vi "set_S12CON.vi"(8 "error in (no error)":errorcluster caption="错误输入（无错误）", 9 "S12CON寄存器设置":T1={"S2传感器上升沿绑定动作"=0, "S2传感器下降沿绑定动作"=1, "S1传感器上升沿绑定动作"=2, "S1传感器下降沿绑定动作"=3} {"S1传感器下降沿绑定动作" items=["无动作，无状态通知"=0, "无动作，有通知"=1, "负向连续运行"=2, "减速直到停止"=3, "紧急停止"=4, "负向相对位移控制"=5, "绝对位置清零"=6, "绝对位置清零+相对位移控制"=7, "换向相对位移控制"=9, "正向连续运行"=10, "绝对位置清零+减速直到停止"=11, "绝对位置清零+紧急停止"=12, "正向相对位移控制"=13, "换向连续运行"=14, "脱机"=15]; "S1传感器上升沿绑定动作" items=["无动作，无状态通知"=0, "无动作，有通知"=1, "负向连续运行"=2, "减速直到停止"=3, "紧急停止"=4, "负向相对位移控制"=5, "绝对位置清零"=6, "绝对位置清零+相对位移控制"=7, "换向相对位移控制"=9, "正向连续运行"=10, "绝对位置清零+减速直到停止"=11, "绝对位置清零+紧急停止"=12, "正向相对位移控制"=13, "换向连续运行"=14, "脱机"=15]; "S2传感器下降沿绑定动作" items=["无动作，无状态通知"=0, "无动作，有通知"=1, "负向连续运行"=2, "减速直到停止"=3, "紧急停止"=4, "负向相对位移控制"=5, "绝对位置清零"=6, "绝对位置清零+相对位移控制"=7, "换向相对位移控制"=9, "正向连续运行"=10, "绝对位置清零+减速直到停止"=11, "绝对位置清零+紧急停止"=12, "正向相对位移控制"=13, "换向连续运行"=14, "脱机"=15]; "S2传感器上升沿绑定动作" items=["无动作，无状态通知"=0, "无动作，有通知"=1, "负向连续运行"=2, "减速直到停止"=3, "紧急停止"=4, "负向相对位移控制"=5, "绝对位置清零"=6, "绝对位置清零+相对位移控制"=7, "换向相对位移控制"=9, "正向连续运行"=10, "绝对位置清零+减速直到停止"=11, "绝对位置清零+紧急停止"=12, "正向相对位移控制"=13, "换向连续运行"=14, "脱机"=15]}, 11 "StepMotor输入":refnum<class "StepMotor.lvclass">) -> (0 "error out":errorcluster caption="错误输出", 3 "StepMotor输出":refnum<class "StepMotor.lvclass">)   [LabVIEW 2016, in "MotionControl_UFO_3DOF.lvlib" / "StepMotor.lvclass"]
uses:
  <userlib>/MotionControl_UFO_3DOF/StepMotor/StepMotor.lvclass
  <userlib>/MotionControl_UFO_3DOF/StepMotor/S12CON.ctl
  <userlib>/MotionControl_UFO_3DOF/StepMotor/StepMotor.lvclass/StepMotor.ctl
  <userlib>/UISimCanFunc_wrapper/UISimCanFunc_wrapper.lvlib
panel:
  out "function return":u32
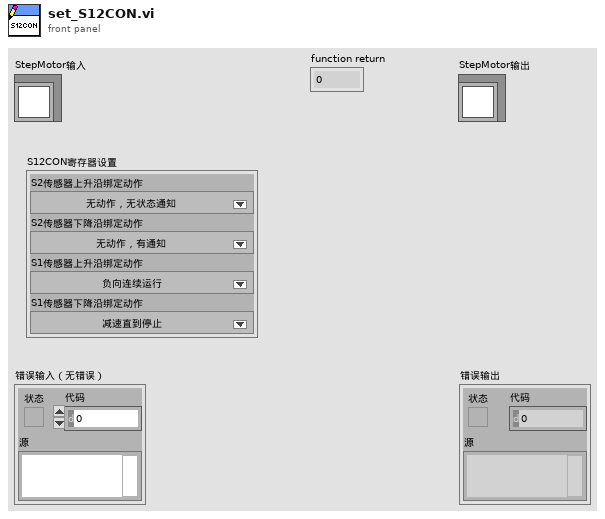
[diagram p1: front panel]
types:
  T1 = typedef "MotionControl_UFO_3DOF.lvlib/StepMotor.lvclass/S12CON.ctl" = cluster{"S2传感器上升沿绑定动作":u32, "S2传感器下降沿绑定动作":u32, "S1传感器上升沿绑定动作":u32, "S1传感器下降沿绑定动作":u32}
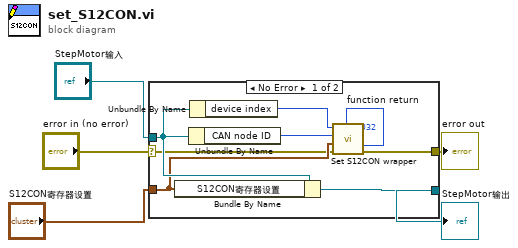
[diagram p0: block diagram]
diagram:
  n1 = case shown="No Error" "error in (no error)" {
    selector: "error in (no error)" -> [w7 w14]
    tunnel: [w11 w14] -> w4
    tunnel: [w13 w15] -> w2
    tunnel: "StepMotor输入" -> [w12 w15]
    tunnel: "S12CON寄存器设置" -> [w8 _]
    frame No Error {
      n2 = Bundle By Name(cluster=w12, "S12CON寄存器设置"=w8) -> (w13:refnum<class "StepMotor.lvclass">)
      n3 = Unbundle By Name(w12) -> ("CAN node ID"=w9:u32)
      n4 = Unbundle By Name(w12) -> ("device index"=w10:u32)
      n5 = call <userlib>:"Set S12CON wrapper.vi"("error in (no error)"=w7, "pS12ConIn"=w8, "dwCanNodeId"=w9, "dwDevIndex"=w10) -> ("error out"=w11:errorcluster, "function return"=→"function return":u32)  [unwired: 5 in, 1 out]
    }
    frame Error {
    }
  }
  "error out" <- w4
  "StepMotor输出" <- w2
